vi "calc number of zernike coefficients.vi"(10 "Zernicke Order":i32, 11 "Array Zernike um":sgl[](array[numeric])) -> (3 "ZernikeCoeffs":sgl[](array[numeric]))   [LabVIEW 2020, in "ThorlabsWFS.lvclass"]
uses:
  ThorlabsWFS.lvclass
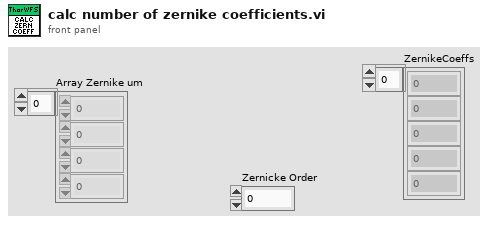
[diagram p1: front panel]
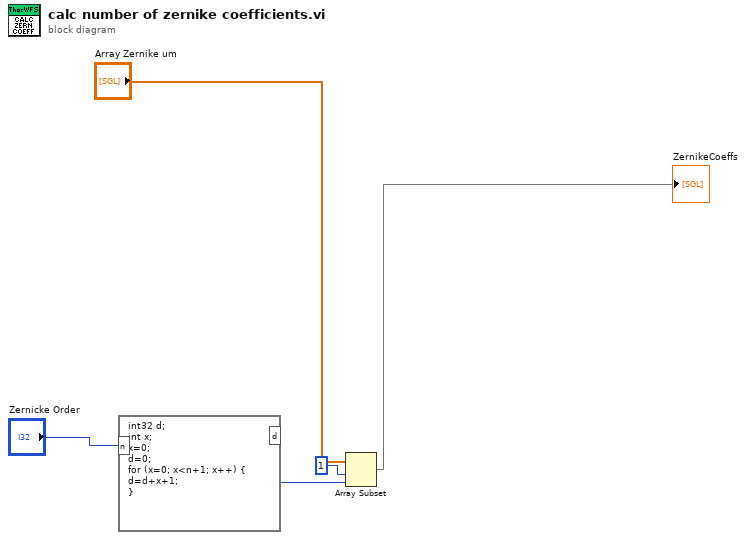
[diagram p0: block diagram]
diagram:
  n1 = formula code="int32 d;\nint x;\nx=0;\nd=0;\nfor (x=0; x<n+1; x++) {\nd=d+x+1;\n}"("n"="Zernicke Order") -> ("d"=w2:i32)
  n2 = Array Subset(array="Array Zernike um", index=1, length=w2) -> (→"ZernikeCoeffs":sgl[])
